vi "PNA_configure.vi"(2 "error in (no error)":errorcluster, 3 "PNA_control":T1={"Channel (1)"=1, "Start Frequency (Hz)"=1000000.0, "Stop Frequency (Hz)"=10000000000.0, "Sweep Points (201)"=201, "Sweep Type (0: Linear)"=0, "Sweep Generation (1: Analog)"=1, "Bandwidth (Hz)"=100000.0, "Average Count (1)"=1, "Enable Average "=FALSE, "Power"={"Attenuation (0 dB)"=0.0, "Power Level (0 dBm)"=0.0, "Enable Auto Attenuation"=TRUE, "Enable RF Power"=TRUE, "Enable Power Slope"=FALSE, "Port (1)"=1, "Power Slope (0 dB/GHz)"=0.0}, "Enable Reduce IF Bandwidth "=TRUE, "Electrical delay"={"Unit (0: Meter)"=0, "Waveguide Cutoff Frequency (Hz)"=45000000.0, "Distance (0)"=0.0, "Medium "=0, "Delay (0 s)"=0.0}, "Measurement name"=[], "Measurement Parameters (S11)"=[]} {"Electrical delay"."Medium" items=["Coaxial", "Waveguide"]; "Electrical delay"."Unit (0: Meter)" items=["Meter", "Feet", "Inch"]; "Sweep Generation (1: Analog)" items=["Stepped", "Analog"]; "Sweep Type (0: Linear)" items=["Linear", "Logarithmic", "Power", "CW", "Segment", "Phase"]}, 4 "PNA_visa":refnum<visa-resource-name>) -> (0 "error out":errorcluster, 1 "PNA_visa_out":refnum<visa-resource-name>)   [LabVIEW 2020]
uses:
  <instrlib>/Keysight PNA Series/Keysight PNA Series.lvlib
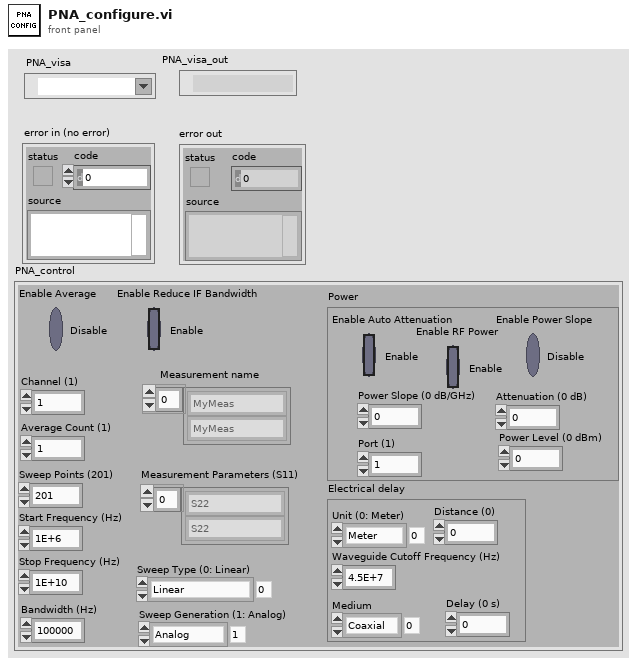
[diagram p1: front panel]
types:
  T1 = cluster{"Channel (1)":i32, "Start Frequency (Hz)":dbl, "Stop Frequency (Hz)":dbl, "Sweep Points (201)":i32, "Sweep Type (0: Linear)":i32, "Sweep Generation (1: Analog)":i32, "Bandwidth (Hz)":dbl, "Average Count (1)":i32, "Enable Average ":bool, "Power":cluster{"Attenuation (0 dB)":dbl, "Power Level (0 dBm)":dbl, "Enable Auto Attenuation":bool, "Enable RF Power":bool, "Enable Power Slope":bool, "Port (1)":i32, "Power Slope (0 dB/GHz)":dbl}, "Enable Reduce IF Bandwidth ":bool, "Electrical delay":cluster{"Unit (0: Meter)":i32, "Waveguide Cutoff Frequency (Hz)":dbl, "Distance (0)":dbl, "Medium ":i32, "Delay (0 s)":dbl}, "Measurement name":string[], "Measurement Parameters (S11)":string[]}
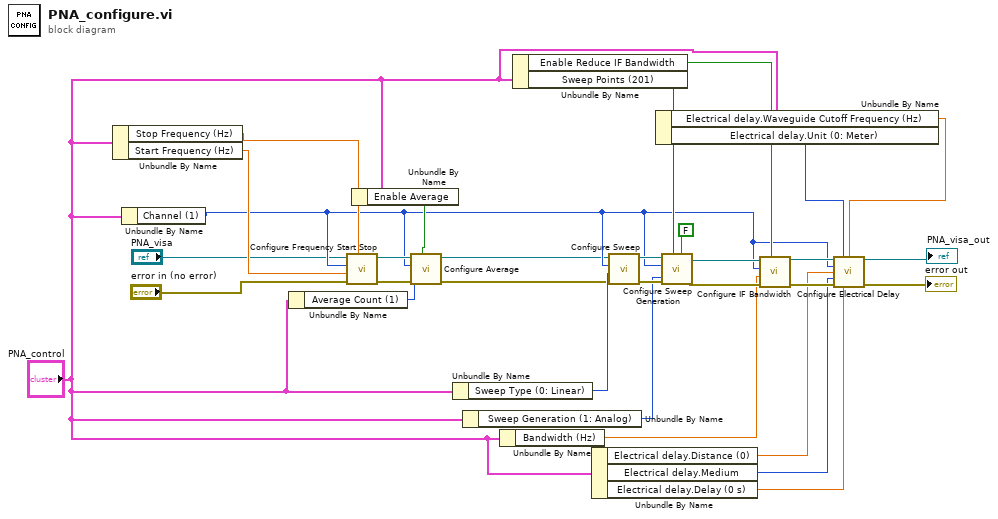
[diagram p0: block diagram]
diagram:
  n1 = Unbundle By Name("PNA_control") -> ("Stop Frequency (Hz)"=w25:dbl, "Start Frequency (Hz)"=w26:dbl)
  n2 = Unbundle By Name("PNA_control") -> ("Channel (1)"=w5:i32)
  n3 = Unbundle By Name("PNA_control") -> ("Average Count (1)"=w18:i32)
  n4 = call <instrlib>:"Configure Frequency Start Stop.vi"("Stop Frequency (2E+6 Hz)"=w25, "error in (no error)"="error in (no error)", "Start Frequency (1E+6 Hz)"=w26, "Channel (1)"=w5, "VISA resource name"="PNA_visa") -> ("error out"=w19:errorcluster, "VISA resource name out"=w20:refnum<visa-resource-name>)  [unwired: 5 in]
  n5 = Unbundle By Name("PNA_control") -> ("Enable Average"=w17:bool)
  n6 = call <instrlib>:"Configure Average.vi"("Enable Average (F: Disable)"=w17, "error in (no error)"=w19, "Average Count (1)"=w18, "Channel (1)"=w5, "VISA resource name"=w20) -> ("error out"=w2:errorcluster, "VISA resource name out"=w1:refnum<visa-resource-name>)  [unwired: 5 in]
  n7 = Unbundle By Name("PNA_control") -> ("Sweep Type (0: Linear)"=w23:i32)
  n8 = Unbundle By Name("PNA_control") -> ("Sweep Generation (1: Analog)"=w22:i32)
  n9 = Unbundle By Name("PNA_control") -> ("Bandwidth (Hz)"=w21:dbl)
  n10 = Unbundle By Name("PNA_control") -> ("Enable Reduce IF Bandwidth"=w14:bool, "Sweep Points (201)"=w24:i32)
  n11 = Unbundle By Name("PNA_control") -> ("Electrical delay.Distance (0)"=w8:dbl, "Electrical delay.Medium"=w7:i32, "Electrical delay.Delay (0 s)"=w6:dbl)
  n12 = call <instrlib>:"Configure Sweep.vi"("error in (no error)"=w2, "Sweep Type (0: Linear)"=w23, "Channel (1)"=w5, "VISA resource name"=w1) -> ("error out"=w31:errorcluster, "VISA resource name out"=w30:refnum<visa-resource-name>)  [unwired: 6 in]
  n13 = Unbundle By Name("PNA_control") -> ("Electrical delay.Waveguide Cutoff Frequency (Hz)"=w11:dbl, "Electrical delay.Unit (0: Meter)"=w10:i32)
  n14 = call <instrlib>:"Configure Sweep Generation.vi"("Auto Sweep or Dwell Time (T: Enable)"=FALSE ("Enable Auto Sweep/Dwell Time (T: Enable)"), "Sweep Generation (1: Analog)"=w22, "Sweep Points (201)"=w24, "error in (no error)"=w31, "Channel (1)"=w5, "VISA resource name"=w30) -> ("error out"=w28:errorcluster, "VISA resource name out"=w27:refnum<visa-resource-name>)  [unwired: 4 in]
  n15 = call <instrlib>:"Configure IF Bandwidth.vi"("Enable Reduce IF Bandwidth (T: Enable)"=w14, "error in (no error)"=w28, "Bandwidth (100000 Hz)"=w21, "Channel (1)"=w5, "VISA resource name"=w27) -> ("error out"=w15:errorcluster, "VISA resource name out"=w16:refnum<visa-resource-name>)  [unwired: 5 in]
  n16 = call <instrlib>:"Configure Electrical Delay.vi"("VISA resource name"=w16, "Unit (0: Meter)"=w10, "Waveguide Cutoff Frequency (4.5E+7 Hz)"=w11, "Channel (1)"=w5, "Distance (0)"=w8, "Medium (0: Coaxial)"=w7, "error in (no error)"=w15, "Delay (0 s)"=w6) -> ("VISA resource name out"=→"PNA_visa_out":refnum<visa-resource-name>, "error out"=→"error out":errorcluster)  [unwired: 6 in]
